vi "configure_version.vi"(8 "error in (no error)":errorcluster, 11 "lv-build-default in":refnum<class "lv-builder.lvclass">) -> (0 "error out":errorcluster, 3 "lv-build-default out":refnum<class "lv-builder.lvclass">)   [LabVIEW 2015, in "lv-builder.lvclass"]
uses:
  lv-builder.lvclass
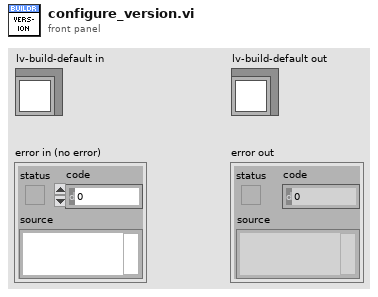
[diagram p1: front panel]
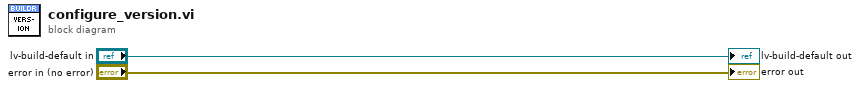
[diagram p0: block diagram]
diagram:
  "error out" <- "error in (no error)"
  "lv-build-default out" <- "lv-build-default in"
